vi "Dropper.vi"(8 "error in (no error)":errorcluster, 10 "point(x,y)":cluster{"x":i16, "y":i16}, 11 "Data in":T1={"Class"={"Ants"=refnum, "Layer"=refnum, "Templates"=refnum, "Icon"=refnum, "Glyph"=refnum, "Settings"=refnum, "Tools"=refnum, "History"=refnum}, "Ref"={"Add Layer"=refnum, "Remove Layer"=refnum, "Line Text"=[], "Body Text Spec"=refnum, "DNL_Font"=refnum, "glyph path str"=refnum, "templates path str"=refnum, "Arrow Up"=refnum, "Arrow Down"=refnum, "IE VI Ref"=refnum, "Glyphs tree"=refnum, "Templates tree"=refnum, "Layer Icon Text"=refnum, "Layer Template"=refnum, "Body Text"=refnum, "Search Templates"=refnum, "TextMarker"=refnum, "Tab Control"=refnum, "Search Glyphs"=refnum, "Line Color"=refnum, "DNL_Glyphs []"=refnum, "Fill Color"=refnum, "Tools"=refnum, "Icon"=refnum, "Preview"=refnum, "Ants"=refnum, "Terminals"=refnum, "menu reference"=refnum, "LayerNames"=[], "GlyphLoadAnimation"=refnum, "TemplateLoadAnimation"=refnum, "refreshGlyphs"=refnum, "refreshTemplates"=refnum}, "Support"={"AntsRect"={"left"=0, "top"=0, "right"=0, "bottom"=0}, "Mouse Move Coords"={"Horizontal"=0, "Vertical"=0}, "Mouse Down Coords"={"Horizontal"=0, "Vertical"=0}, "Temp Coord"={"Horizontal"=0, "Vertical"=0}, "Action"=enum."Default", "Edge Color"=4914962, "Fill Color"=16860, "Mouse Down?"=FALSE, "Draft Mode?"=FALSE, "Temp Icon"=bytes[3102], "CTRL Pressed"=FALSE, "Move Selection?"=FALSE, "AntsRect Orig"={"left"=0, "top"=0, "right"=0, "bottom"=0}, "Text"="", "TM Set?"=FALSE, "Mouse inside icon?"=FALSE, "Tool (old value)"=0, "Pencil Move Color"=0, "Swap Colors?"=FALSE, "Shift pressed?"=FALSE}}) -> (0 "error out":errorcluster, 2 "Color":u32, 3 "Data out":T1={"Class"={"Ants"=refnum, "Layer"=refnum, "Templates"=refnum, "Icon"=refnum, "Glyph"=refnum, "Settings"=refnum, "Tools"=refnum, "History"=refnum}, "Ref"={"Add Layer"=refnum, "Remove Layer"=refnum, "Line Text"=[], "Body Text Spec"=refnum, "DNL_Font"=refnum, "glyph path str"=refnum, "templates path str"=refnum, "Arrow Up"=refnum, "Arrow Down"=refnum, "IE VI Ref"=refnum, "Glyphs tree"=refnum, "Templates tree"=refnum, "Layer Icon Text"=refnum, "Layer Template"=refnum, "Body Text"=refnum, "Search Templates"=refnum, "TextMarker"=refnum, "Tab Control"=refnum, "Search Glyphs"=refnum, "Line Color"=refnum, "DNL_Glyphs []"=refnum, "Fill Color"=refnum, "Tools"=refnum, "Icon"=refnum, "Preview"=refnum, "Ants"=refnum, "Terminals"=refnum, "menu reference"=refnum, "LayerNames"=[], "GlyphLoadAnimation"=refnum, "TemplateLoadAnimation"=refnum, "refreshGlyphs"=refnum, "refreshTemplates"=refnum}, "Support"={"AntsRect"={"left"=0, "top"=0, "right"=0, "bottom"=0}, "Mouse Move Coords"={"Horizontal"=0, "Vertical"=0}, "Mouse Down Coords"={"Horizontal"=0, "Vertical"=0}, "Temp Coord"={"Horizontal"=0, "Vertical"=0}, "Action"=enum."Default", "Edge Color"=4914962, "Fill Color"=16860, "Mouse Down?"=FALSE, "Draft Mode?"=FALSE, "Temp Icon"=bytes[3102], "CTRL Pressed"=FALSE, "Move Selection?"=FALSE, "AntsRect Orig"={"left"=0, "top"=0, "right"=0, "bottom"=0}, "Text"="", "TM Set?"=FALSE, "Mouse inside icon?"=FALSE, "Tool (old value)"=0, "Pencil Move Color"=0, "Swap Colors?"=FALSE, "Shift pressed?"=FALSE}})   [LabVIEW 2020, in "Tools Paint.lvclass"]
uses:
  Tools Paint.lvclass
  Ants/Ants.lvclass
  FakedArray/FakedArray.lvclass
  vi.lib/LabVIEW Icon API/lv_icon/Classes/Icon/Icon.lvclass
  Icon Library/Glyph.lvclass
  Settings/Settings.lvclass
  History/History/History.lvclass
  vi.lib/LabVIEW Icon API/lv_icon/Classes/Icon Framework/Icon Framework.lvclass
  vi.lib/LabVIEW Icon API/lv_icon/Classes/Layer/Layer.lvclass
  Tools Paint.lvclass/Tools Paint.ctl
  vi.lib/LabVIEW Icon API/LabVIEW Icon API.lvlib
  lv_icon.lvlib
  <vilib>/Utility/miscctls.llb/LVPoint32TypeDef.ctl
  Controls/SupportClass_Action.ctl
  vi.lib/LabVIEW Icon API/lv_icon/Controls/IEColor.ctl
  Controls/Support Cluster.ctl
  Controls/References Cluster.ctl
  Controls/IE Classes.ctl
  Controls/Global Data.ctl
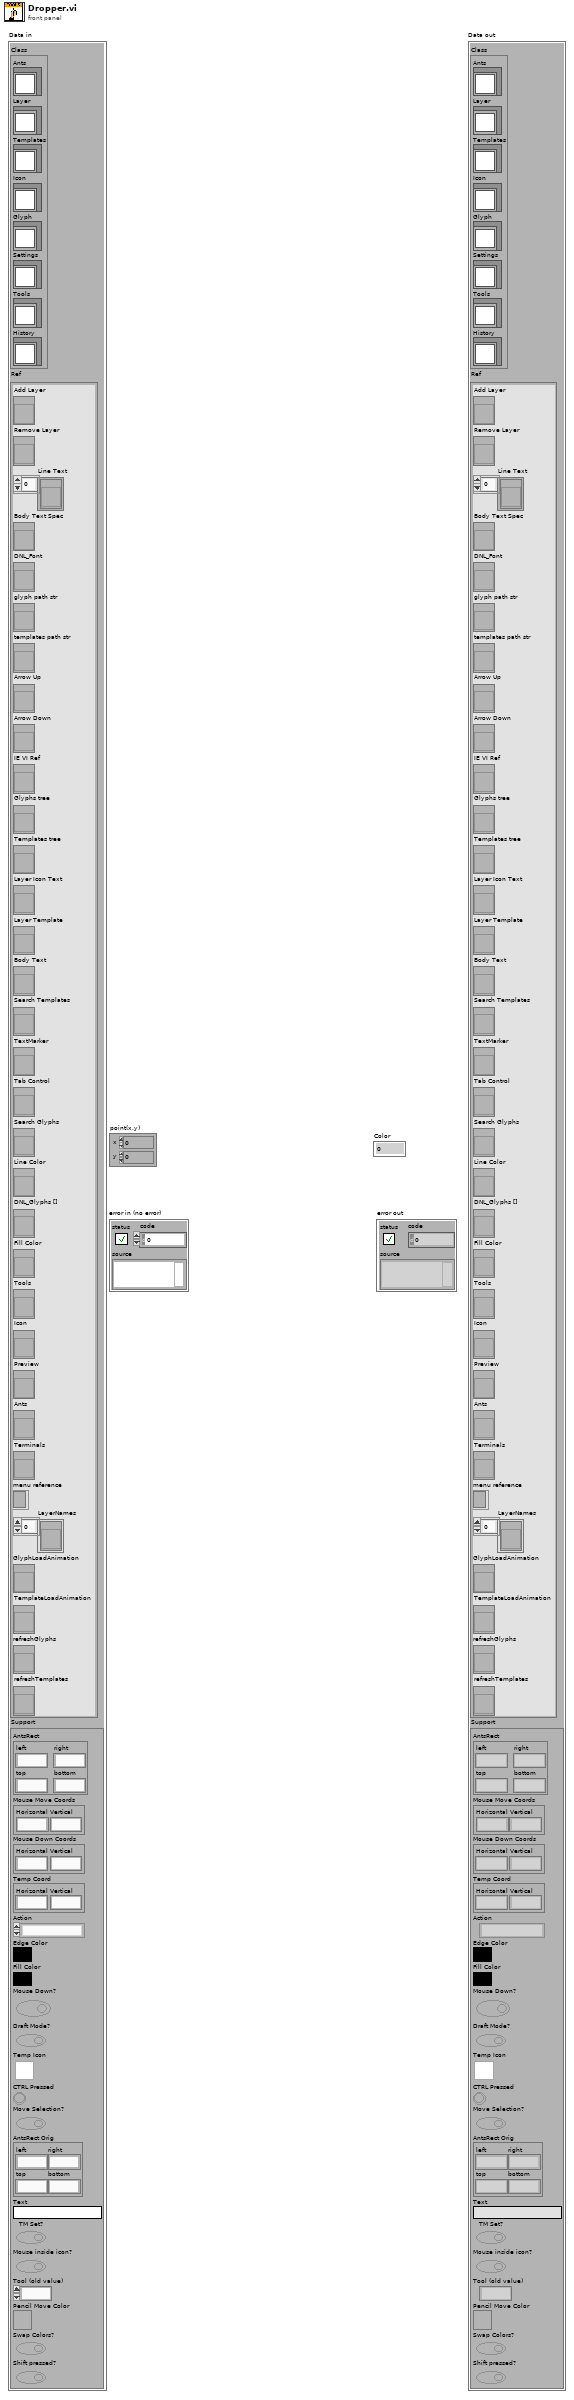
[diagram p1: front panel]
types:
  T1 = typedef "lv_icon.lvlib/Global Data.ctl" = cluster{"Class":T2, "Ref":T3, "Support":T4}
  T2 = typedef "lv_icon.lvlib/IE Classes.ctl" = cluster{"Ants":refnum<class "Ants.lvclass">, "Layer":refnum<class "FakedArray.lvclass">, "Templates":refnum<class "FakedArray.lvclass">, "Icon":refnum<class "Icon.lvclass">, "Glyph":refnum<class "Glyph.lvclass">, "Settings":refnum<class "Settings.lvclass">, "Tools":refnum<class "Tools Paint.lvclass">, "History":refnum<class "History.lvclass">}
  T3 = typedef "lv_icon.lvlib/References Cluster.ctl" = cluster{"Add Layer":refnum<vi>, "Remove Layer":refnum<vi>, "Line Text":refnum<vi>[], "Body Text Spec":refnum<vi>, "DNL_Font":refnum<vi>, "glyph path str":refnum<vi>, "templates path str":refnum<vi>, "Arrow Up":refnum<vi>, "Arrow Down":refnum<vi>, "IE VI Ref":refnum<vi>, "Glyphs tree":refnum<vi>, "Templates tree":refnum<vi>, "Layer Icon Text":refnum<vi>, "Layer Template":refnum<vi>, "Body Text":refnum<vi>, "Search Templates":refnum<vi>, "TextMarker":refnum<vi>, "Tab Control":refnum<vi>, "Search Glyphs":refnum<vi>, "Line Color":refnum<vi>, "DNL_Glyphs []":refnum<vi>, "Fill Color":refnum<vi>, "Tools":refnum<vi>, "Icon":refnum<vi>, "Preview":refnum<vi>, "Ants":refnum<vi>, "Terminals":refnum<vi>, "menu reference":refnum<k9>, "LayerNames":refnum<vi>[], "GlyphLoadAnimation":refnum<vi>, "TemplateLoadAnimation":refnum<vi>, "refreshGlyphs":refnum<vi>, "refreshTemplates":refnum<vi>}
  T4 = typedef "lv_icon.lvlib/Support Cluster.ctl" = cluster{"AntsRect":cluster{"left":i16, "top":i16, "right":i16, "bottom":i16}, "Mouse Move Coords":T5, "Mouse Down Coords":T5, "Temp Coord":T5, "Action":T6, "Edge Color":T7, "Fill Color":T7, "Mouse Down?":bool, "Draft Mode?":bool, "Temp Icon":picture, "CTRL Pressed":bool, "Move Selection?":bool, "AntsRect Orig":cluster{"left":i16, "top":i16, "right":i16, "bottom":i16}, "Text":string, "TM Set?":bool, "Mouse inside icon?":bool, "Tool (old value)":u32, "Pencil Move Color":u32, "Swap Colors?":bool, "Shift pressed?":bool}
  T5 = typedef "LVPoint32TypeDef.ctl" = cluster{"Horizontal":i32, "Vertical":i32}
  T6 = typedef "SupportClass_Action.ctl" = enum16{"Default", "Move Selection", "Glyph Library", "Tool"}
  T7 = typedef "IEColor.ctl" = u32
  T8 = typedef "Layer.ctl" = cluster{"LayerIcon":picture, "LayerName":string, "Opacity":u8, "Visibility?":bool}
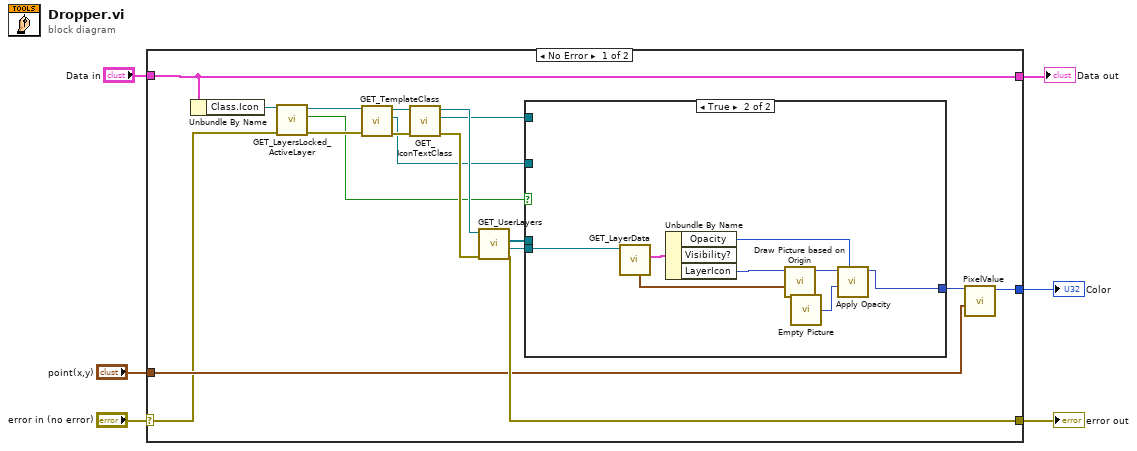
[diagram p0: block diagram]
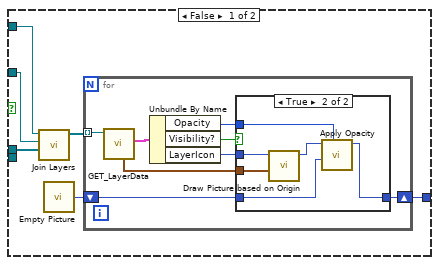
[diagram p2: hidden frame]
diagram:
  n1 = case shown="No Error" "error in (no error)" {
    selector: "error in (no error)" -> [w8 w55]
    tunnel: [w24 w55] -> w5
    tunnel: "point(x,y)" -> [w22 _]
    tunnel: [w21 _] -> w3
    tunnel: "Data in" -> [w7 w54]
    tunnel: [w7 w54] -> w1
    frame No Error {
      n2 = Unbundle By Name(w7) -> ("Class.Icon"=w9:refnum<class "Icon.lvclass">)
      n3 = call-dynamic "GET_LayersLocked_ActiveLayer.vi"("error in (no error)"=w8, "Icon.lvclass in"=w9) -> ("error out"=w15:errorcluster, "Layers Locked?"=w11:bool, "Icon.lvclass out"=w16:refnum<class "Icon.lvclass">)  [unwired: 7 out]
      n4 = call-dynamic "GET_TemplateClass.vi"("error in (no error)"=w15, "Icon.lvclass in"=w16) -> ("error out"=w19:errorcluster, "Icon Framework.lvclass"=w13:refnum<class "Icon Framework.lvclass">, "Icon.lvclass out"=w20:refnum<class "Icon.lvclass">)  [unwired: 7 out]
      n5 = call-dynamic "GET_IconTextClass.vi"("error in (no error)"=w19, "Icon.lvclass in"=w20) -> ("error out"=w17:errorcluster, "Icon Framework.lvclass"=w14:refnum<class "Icon Framework.lvclass">, "Icon.lvclass out"=w18:refnum<class "Icon.lvclass">)  [unwired: 7 out]
      n6 = call-dynamic "GET_UserLayers.vi"("error in (no error)"=w17, "Icon.lvclass in"=w18) -> ("error out"=w24:errorcluster, "Active Layer"=w10:refnum<class "Layer.lvclass">, "All Layers"=w12:refnum<class "Layer.lvclass">[])  [unwired: 7 out]
      n7 = case shown="True" w11 {
        tunnel: [w30 w53] -> w23
        tunnel: w14 -> [w27 _]
        tunnel: w13 -> [w26 _]
        tunnel: w12 -> [w25 _]
        tunnel: w10 -> [_ w46]
        frame False {
          n8 = call "Join Layers.vi"("User Layers"=w25, "Template"=w26, "Icon Text"=w27) -> ("Layer out"=w28:refnum<class "Layer.lvclass">[])  [unwired: 3 in, 5 out]
          n9 = call "Empty Picture"() -> ("empty picture"=w29:picture)
          n10 = for {
            shift-right: [w33] -> w30
            shift-left: w29 -> [w34]
            tunnel: w28 -> [w31] mode=indexing
            n11 = call-dynamic "GET_LayerData.vi"("Layer.lvclass in"=w31) -> ("Data"=w37:T8, "Origin"=w38:T5)  [unwired: 1 in, 8 out]
            n12 = Unbundle By Name(w37) -> ("Opacity"=w35:u8, "Visibility?"=w36:bool, "LayerIcon"=w32:picture)
            n13 = case shown="True" w36 {
              tunnel: w38 -> [_ w45]
              tunnel: w35 -> [_ w44]
              tunnel: w34 -> [w39 w42]
              tunnel: [w39 w41] -> w33
              tunnel: w32 -> [_ w40]
              frame False {
              }
              frame True {
                n14 = call "Draw Picture based on Origin.vi"("Origin"=w45, "LayerIcon in"=w40) -> ("LayerIcon out"=w43:picture)  [unwired: 1 in, 8 out]
                n15 = call "Apply Opacity.vi"("% (100)"=w44, "Bottom"=w42, "Top"=w43) -> ("new picture"=w41:picture)  [unwired: 8 out]
              }
            }
          }
        }
        frame True {
          n16 = call-dynamic "GET_LayerData.vi"("Layer.lvclass in"=w46) -> ("Data"=w50:T8, "Origin"=w51:T5)  [unwired: 1 in, 8 out]
          n17 = Unbundle By Name(w50) -> ("Opacity"=w49:u8, "LayerIcon"=w48:picture)  [unwired: 1 out]
          n18 = call "Draw Picture based on Origin.vi"("Origin"=w51, "LayerIcon in"=w48) -> ("LayerIcon out"=w47:picture)  [unwired: 1 in, 8 out]
          n19 = call "Empty Picture"() -> ("empty picture"=w52:picture)
          n20 = call "Apply Opacity.vi"("% (100)"=w49, "Bottom"=w52, "Top"=w47) -> ("new picture"=w53:picture)  [unwired: 8 out]
        }
      }
      n21 = call "PixelValue.vi"("point(x,y)"=w22, "Picture"=w23) -> ("Color"=w21:u32)  [unwired: 9 out]
    }
    frame Error {
    }
  }
  "error out" <- w5
  "Color" <- w3
  "Data out" <- w1
